vi "LS Durability Main ALTERNATE (FPGA).vi"() -> ()   [LabVIEW 2019]
uses:
  <vilib>/eio/EIONode/EIONode.xnode
  <vilib>/rvi/eio/common/nirviEmuTemplateMethod_errors.vi
  <vilib>/rvi/DataTransferAndStorage/Container/XNode/niFpgaContainer.xnode
  <vilib>/rvi/FIFO/Fifo_Resource/niFpgaFifoEmulationRefIn.vi
panel:
  out "FIFO microseconds":u32
  in  "Subtract Noise":bool
  out "Anomaly Array":fxp<+/-,29,18>[](array[numeric])
  in  "Enable2ndStepCheck":bool
  out "Anomaly Resamples":fxp<+/-,28,17>[](array[numeric])
  in  "Anomaly Threshold":fxp<+/-,28,17>=0.02978515625
  out "Bank2Active":bool
  out "Bank1Active":bool
  out "Bank2On":bool
  out "Bank1On":bool
  in  "Enable Readings":bool[](array[boolean])=[FALSE, FALSE, FALSE, FALSE, FALSE, FALSE, FALSE, FALSE, FALSE, FALSE, FALSE, FALSE]
  in  "Opens Resets":bool[](array[boolean])=[FALSE, FALSE, FALSE, FALSE, FALSE, FALSE, FALSE, FALSE, FALSE, FALSE, FALSE, FALSE]
  in  "Enable Opens":bool[](array[boolean])=[FALSE, FALSE, FALSE, FALSE, FALSE, FALSE, FALSE, FALSE, FALSE, FALSE, FALSE, FALSE]
  out "Opens Detected":u16[](array[numeric])
  out "Opens Loop Time (usec)":u32=1000
  in  "Bank2(Pulse/Const)":bool
  in  "Bank2Const(On/Off)":bool
  out "Anomalies (Last Cycle)":i32[](array[numeric])
  out "Cycle Starts":bool[](array[boolean])
  out "Anomalies (Total)":i32[](array[numeric])
  out "Anomalies/Cycle":i32[](array[numeric])
  in  "Normal Steps":u32=98
  out "Cycles":u32[](array[numeric])
  out "Anomaly Loop Time (usec)":u32=1000
  out "Steps":u32[](array[numeric])
  in  "Step Threshold":fxp<+/-,28,17>=0.02978515625
  in  "Enable Anomalies":bool[](array[boolean])=[FALSE, FALSE, FALSE, FALSE, FALSE, FALSE, FALSE, FALSE, FALSE, FALSE, FALSE, FALSE]
  in  "Anomaly Resets":bool[](array[boolean])=[FALSE, FALSE, FALSE, FALSE, FALSE, FALSE, FALSE, FALSE, FALSE, FALSE, FALSE, FALSE]
  in  "Bank1Const(On/Off)":bool
  in  "Bank1(Pulse/Const)":bool
  in  "PWM Period (Ticks)":u32=4000000
  in  "Duty (Ticks)":i32=2000000
  in  "Invert PWM?":bool=TRUE
  in  "Cycle Resets":bool[](array[boolean])=[FALSE, FALSE, FALSE, FALSE, FALSE, FALSE, FALSE, FALSE, FALSE, FALSE, FALSE, FALSE]
  in  "Points to Avg":i32=20
  in  "Enable Cycles":bool[](array[boolean])=[FALSE, FALSE, FALSE, FALSE, FALSE, FALSE, FALSE, FALSE, FALSE, FALSE, FALSE, FALSE]
  out "Total Cycles":u32[](array[numeric])
  in  "Cycle Threshold":fxp<+/-,28,17>=1.2001953125
  out "AI Avg Loop Time (usec)":u32=1000
  out "Analog Inputs":fxp<+/-,28,17>[](array[numeric])
  out "AI Loop Time (usec)":u32=70
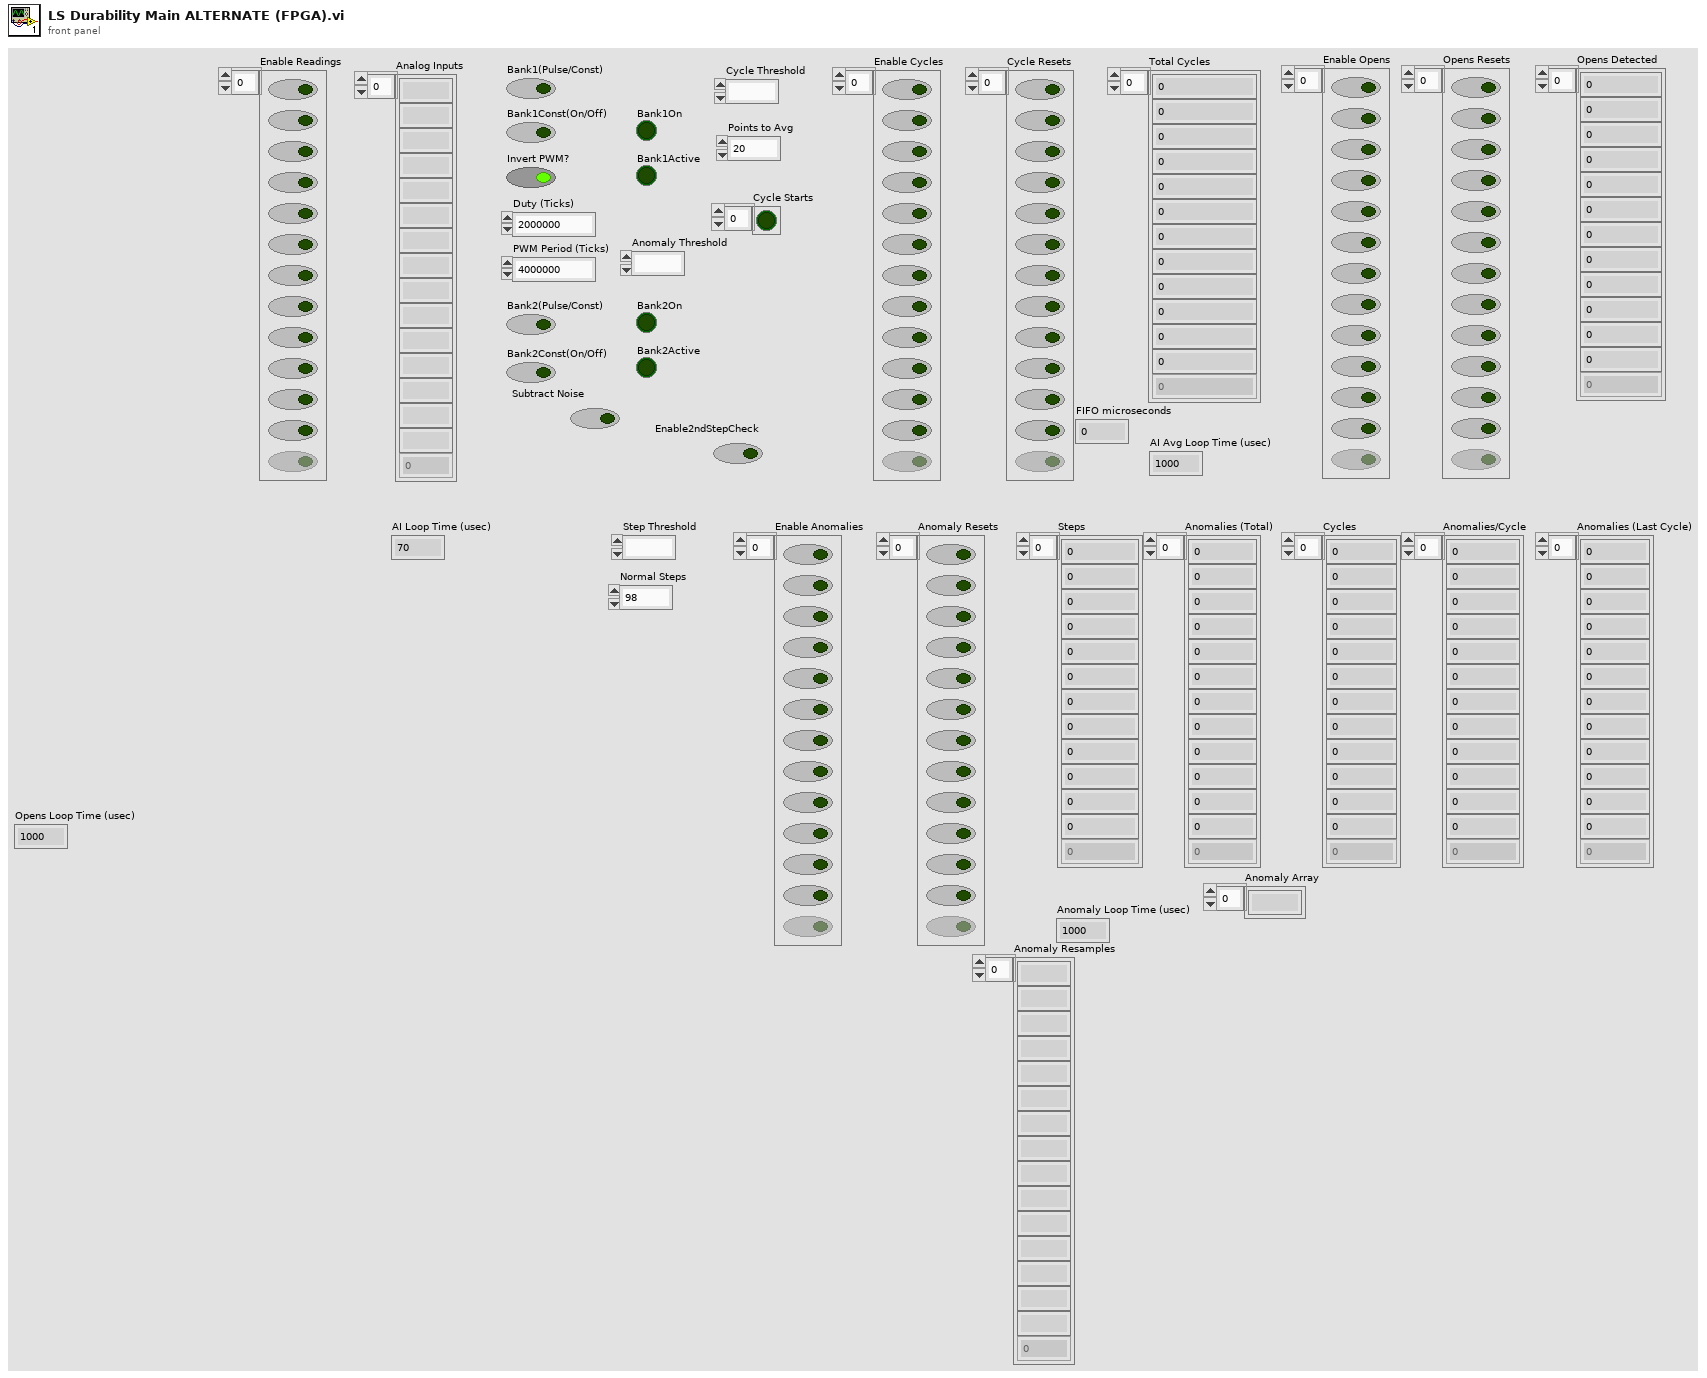
[diagram p1: front panel]
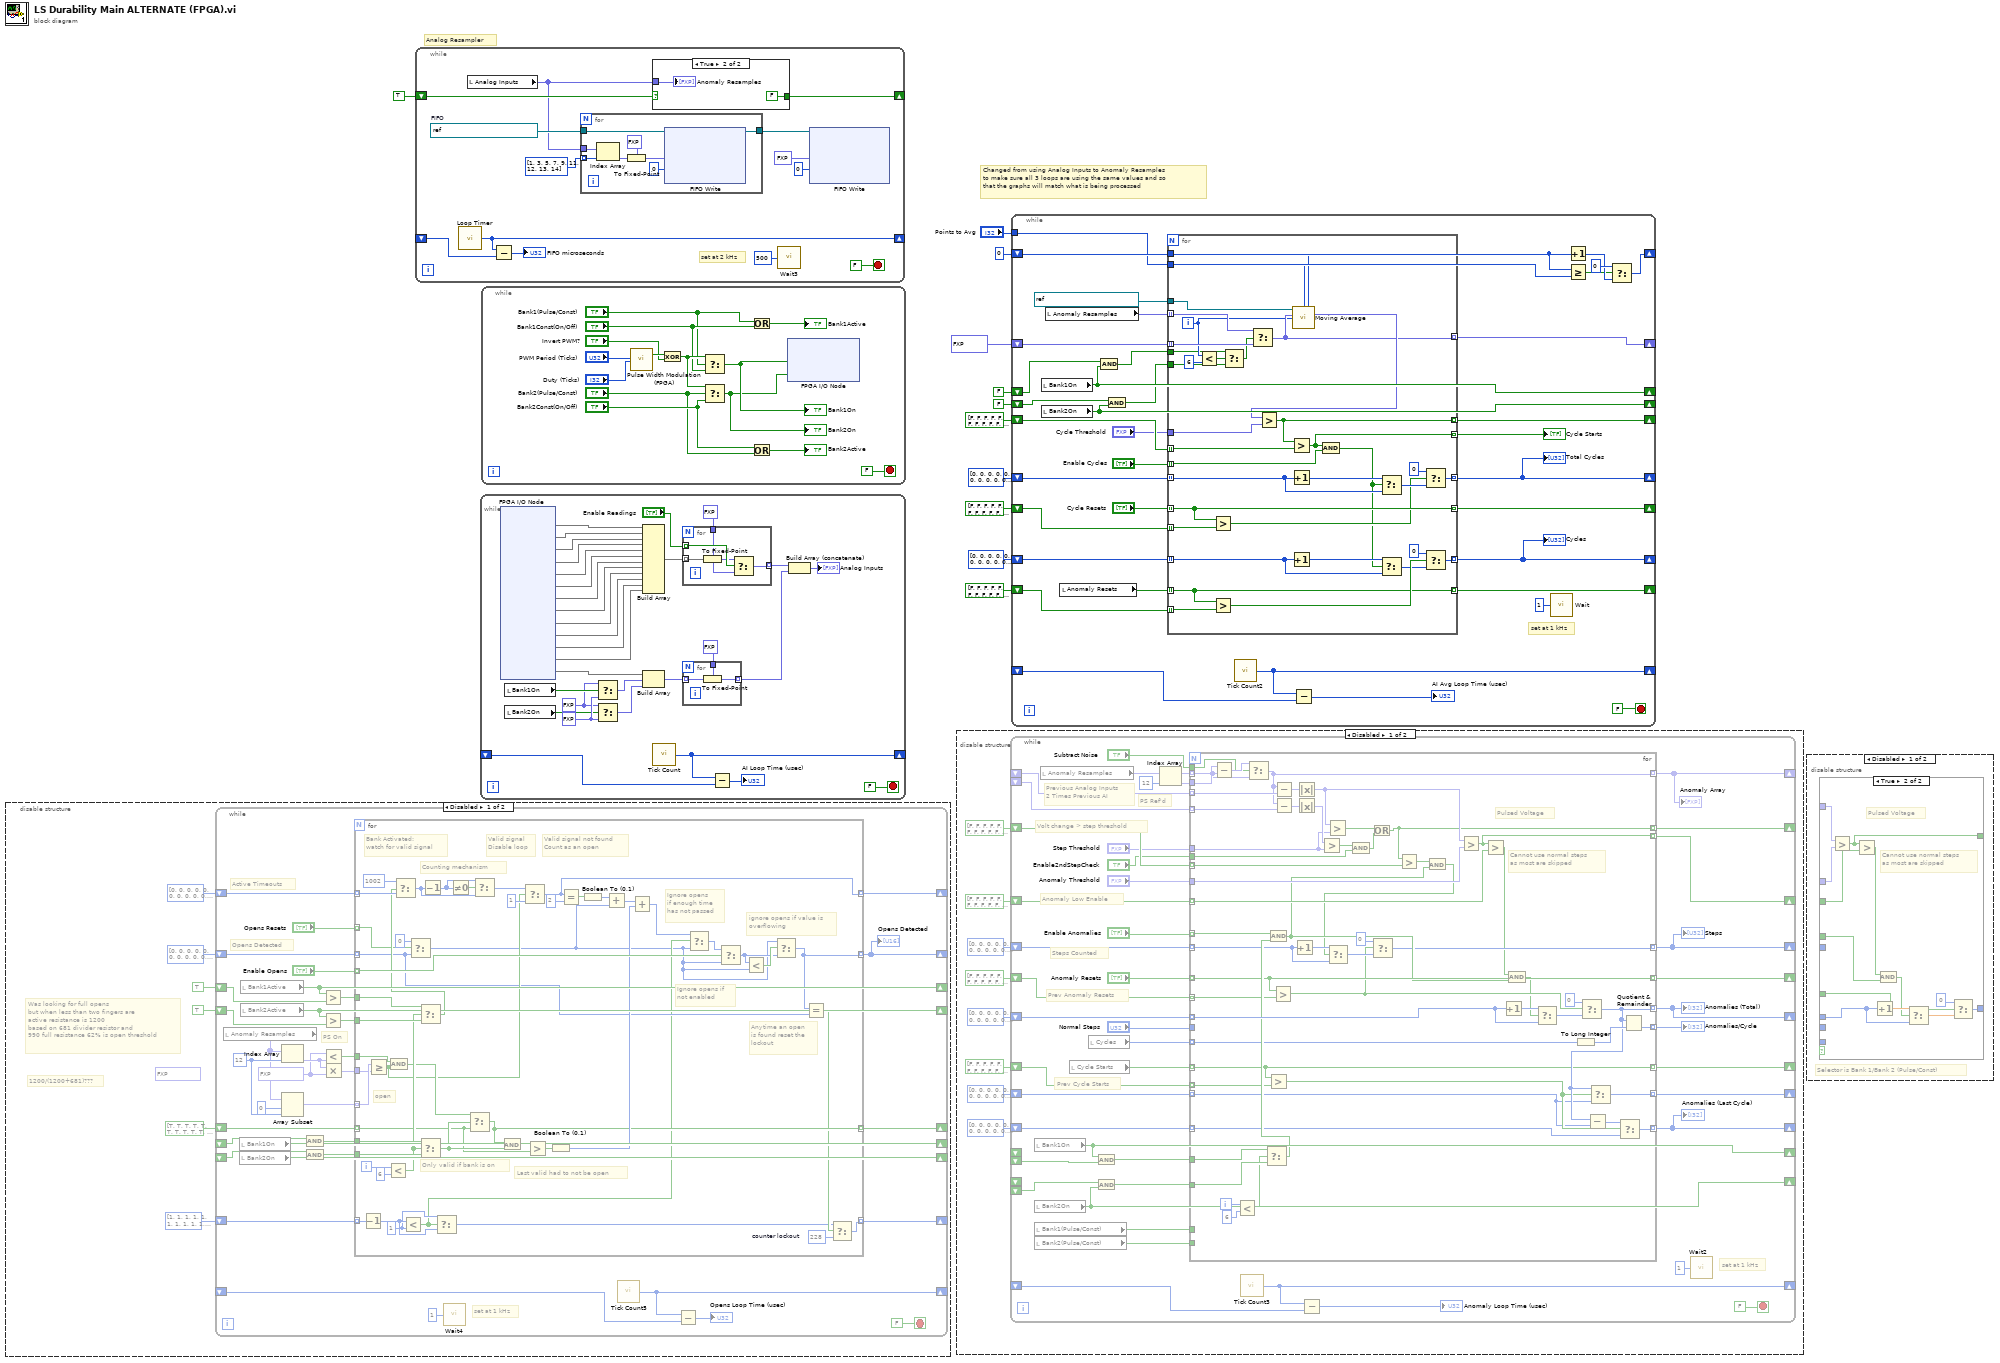
[diagram p0: block diagram]
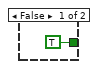
[diagram p4: hidden frame]
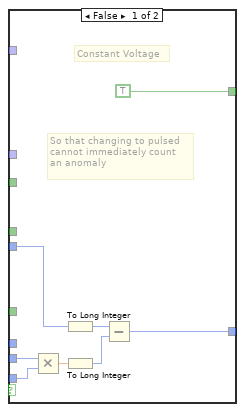
[diagram p5: hidden frame]
diagram:
  # "Changed from using Analog Inputs to Anomaly Resamples\nto make sure all 3 loops are using the same values and so\nthat the graphs will match what is being processed"
  # "Analog Resampler"
  n1 = disable-structure shown="Disabled" {
    frame Disabled {
      (unwired) fxp<+,8,0> 0.94921875
      # "1200/(1200+681)???"
      # "Was looking for full opens\nbut when less than two fingers are\nactive resistance is 1200\nbased on 681 divider resistor and\n990 full resistance 62% is open threshold"
      n2 = while {
        shift-right: [w50] -> _
        shift-left: _ -> [w49]
        shift-right: [w21] -> _
        shift-left: u8[] [0, 0, 0, 0, 0, 0, 0, 0, 0, 0, 0, 0] -> [w45]
        shift-right: [w30] -> _
        shift-left: u16[] [0, 0, 0, 0, 0, 0, 0, 0, 0, 0, 0, 0] -> [w31]
        shift-right: [w37] -> _
        shift-left: bool[] [TRUE, TRUE, TRUE, TRUE, TRUE, TRUE, TRUE, TRUE, TRUE, TRUE, TRUE, TRUE] -> [w36]
        shift-right: [w35] -> _
        shift-left: TRUE ("Bank2Active") -> [w33]
        shift-right: [w34] -> _
        shift-left: TRUE ("Bank1Active") -> [w32]
        shift-right: [w24] -> _
        shift-left: _ -> [w22]
        shift-right: [w25] -> _
        shift-left: _ -> [w23]
        shift-right: [w19] -> _
        shift-left: u16[] [1, 1, 1, 1, 1, 1, 1, 1, 1, 1, 1, 1] -> [w20]
        stop <- FALSE stop-if-true
        w38 = fxp<+,8,0> 0.62109375
        w47 = 12 ("length")
        # "Opens Detected"
        # "Active Timeouts"
        # "PS On"
        # "set at 1 kHz"
        n3 = local read "Anomaly Resamples"() -> (w18:fxp<+/-,28,17>[])
        n4 = local read "Bank1On"() -> (w25:bool)
        n5 = local read "Bank2On"() -> (w24:bool)
        n6 = local read "Bank1Active"() -> (w34:bool)
        n7 = local read "Bank2Active"() -> (w35:bool)
        n8 = Index Array(array=w18, index=w47) -> (element=w39:fxp<+/-,28,17>)
        n9 = Array Subset(array=w18, index=0, length=w47) -> (w40:fxp<+/-,28,17>[])
        n10 = And(x=w23, y=w25) -> (x .and. y?=w27:bool)
        n11 = And(x=w22, y=w24) -> (x .and. y?=w26:bool)
        n12 = Greater?(x=w34, y=w32) -> (0:w44:bool)
        n13 = Greater?(x=w35, y=w33) -> (0:w43:bool)
        n14 = Less?(x=w38, y=w39) -> (x < y?=w42:bool)
        n15 = Multiply(x=w39, y=w38) -> (x*y=w41:fxp<+/-,36,17>)
        n16 = for {
          tunnel: w27 -> [w99]
          tunnel: w26 -> [w98]
          tunnel: w44 -> [w96]
          tunnel: w43 -> [w97]
          tunnel: w45 -> [w57] mode=indexing
          tunnel: w31 -> [w84] mode=indexing
          tunnel: "Opens Resets" -> [w68] mode=indexing
          tunnel: "Enable Opens" -> [w82] mode=indexing
          tunnel: [w58] -> w21 mode=indexing
          tunnel: w41 -> [w79]
          tunnel: w40 -> [w80] mode=indexing
          tunnel: w42 -> [w78]
          tunnel: [w69] -> w37 mode=indexing
          tunnel: w36 -> [w74] mode=indexing
          tunnel: [w72] -> w30 mode=indexing
          tunnel: w20 -> [w63] mode=indexing
          tunnel: [w59] -> w19 mode=indexing
          i -> [w101]
          w60 = u16 228  # counter lockout
          w64 = u16 1 ("y")
          # "Ignore opens if\nnot enabled"
          # "Ignore opens\nif enough time\nhas not passed"
          # "Anytime an open\nis found reset the\nlockout"
          # "ignore opens if value is\noverflowing"
          # "Last valid had to not be open"
          # "Only valid if bank is on"
          # "open"
          # "Valid signal not found\nCount as an open"
          # "Valid signal\nDisable loop"
          # "Counting mechanism"
          # "Bank Activated:\nwatch for valid signal"
          n17 = Decrement(x=w63) -> (x-1=w65:u16)
          n18 = Greater Or Equal?(x=w80, y=w79) -> (x >= y?=w71:bool)
          n19 = Less?(x=w101, y=6) -> (x < y?=w95:bool)
          n20 = And(x=w78, y=w71) -> (x .and. y?=w77:bool)
          n21 = Less?(x=w65, y=w64) -> (x < y?=w54:bool)
          n22 = Select(t=u16 0, s=w68, f=w57) -> (s? t:f=w53:u16)
          n23 = Select(t=w96, s=w95, f=w97) -> (s? t:f=w81:bool)
          n24 = Select(t=u16 1002, s=w81, f=w84) -> (s? t:f=w83:u16)
          n25 = Select(t=w99, s=w95, f=w98) -> (s? t:f=w76:bool)
          n26 = Decrement(x=w83) -> (x-1=w88:u16)
          n27 = Select(t=w64, s=w54, f=w65) -> (s? t:f=w61:u16)
          n28 = Not Equal To 0?(x=w88) -> (x != 0?=w87:bool)
          n29 = Select(t=w77, s=w76, f=w74) -> (s? t:f=w69:bool)
          n30 = Select(t=w88, s=w87, f=w83) -> (s? t:f=w89:u16)
          n31 = And(x=w69, y=w76) -> (x .and. y?=w70:bool)
          n32 = Select(t=w89, s=w71, f=u16 1) -> (s? t:f=w72:u16)
          n33 = Greater?(x=w70, y=w74) -> (0:w75:bool)
          n34 = Boolean To (0,1)(Boolean=w75) -> (0, 1=w73:i16)
          n35 = Equal?(x=w72, y=u16 2) -> (x = y?=w91:bool)
          n36 = Boolean To (0,1)(Boolean=w91) -> (0, 1=w92:i16)
          n37 = Add(x=w92, y=w53) -> (x+y=w93:u16)
          n38 = Add(x=w93, y=w73) -> (x+y=w55:u16)
          n39 = Select(t=w55, s=w54, f=w53) -> (s? t:f=w56:u16)
          n40 = Select(t=w56, s=w82, f=w53) -> (s? t:f=w66:u16)
          n41 = Less?(x=w66, y=w53) -> (x < y?=w67:bool)
          n42 = Select(t=w53, s=w67, f=w66) -> (s? t:f=w58:u16)
          n43 = Equal?(x=w58, y=w57) -> (x = y?=w62:bool)
          n44 = Select(t=w61, s=w62, f=w60) -> (s? t:f=w59:u16)
        }
        "Opens Detected" <- w21
        n45 = call "Wait4"("Count(mSec)"=u32 1) -> ()  [unwired: 1 out]
        n46 = call "Tick Count5"() -> ("Tick Count(uSec)"=w50:u32)
        n47 = Subtract(x=w50, y=w49) -> (x-y=→"Opens Loop Time (usec)":u32)
      }
    }
    frame Enabled {
    }
  }
  n48 = while {
    shift-right: [w113] -> _
    shift-left: TRUE -> [w111]
    shift-right: [w105] -> _
    shift-left: _ -> [w104]
    stop <- FALSE stop-if-true
    w110 = refnum<k21> "One Hour Analog Data"  # FIFO
    # "set at 2 kHz"
    n49 = call "Loop Timer"() -> ("Tick Count(uSec)"=w105:u32)  [unwired: 1 in]
    n50 = local read "Analog Inputs"() -> (w109:fxp<+/-,28,17>[])
    n51 = Subtract(x=w105, y=w104) -> (x-y=→"FIFO microseconds":u32)
    n52 = for {
      tunnel: w110 -> [w122]
      tunnel: w109 -> [w117]
      tunnel: [w118] -> w108
      tunnel: i32[] [1, 3, 5, 7, 9, 11, 12, 13, 14] -> [w115] mode=indexing
      n53 = Index Array(array=w117, index=w115) -> (element=w116:fxp<+/-,28,17>)
      n54 = To Fixed-Point(fixed-point type=fxp<+/-,18,5> 0.0 ("AI0"), number=w116) -> (fixed-point=w121:fxp<+/-,18,5>)
      n55 = xnode ("FIFO Write")("Element"=w121, "Timeout"=0, "FIFO In"=w122) -> ("FIFO Out"=w118:refnum<k21>)  [unwired: 1 out]
    }
    n56 = case shown="True" w111 {
      tunnel: w109 -> [_ w125]
      tunnel: [TRUE FALSE] -> w113
      frame False {
      }
      frame True {
        "Anomaly Resamples" <- w125
      }
    }
    n57 = call "Wait3"("Count(uSec)"=u32 500 ("Count(mSec)")) -> ()  [unwired: 1 out]
    n58 = xnode ("FIFO Write")("Element"=fxp<+/-,18,5> -15.0 ("AI0"), "Timeout"=0, "FIFO In"=w108) -> ()  [unwired: 2 out]
  }
  n59 = while {
    shift-right: [w155] -> _
    shift-left: _ -> [w154]
    stop <- FALSE stop-if-true
    w128 = fxp<+/-,24,5> 1.0 ("AI13")
    w131 = fxp<+/-,24,5> 0.0 ("AI13")
    n60 = xnode "FPGA I/O Node"() -> ("AI0"=w152, "AI1"=w151, "AI2"=w150, "AI3"=w149, "AI4"=w148, "AI5"=w147, "AI6"=w146, "AI7"=w145, "AI8"=w144, "AI9"=w143, "AI10"=w142, "AI11"=w141, "AI12"=w138)  [unwired: 13 in, 13 out]
    n61 = local read "Bank1On"() -> (w130:bool)
    n62 = local read "Bank2On"() -> (w129:bool)
    n63 = Select(t=w128, s=w130, f=w131) -> (s? t:f=w127:fxp<+/-,24,5>)
    n64 = Select(t=w128, s=w129, f=w131) -> (s? t:f=w126:fxp<+/-,24,5>)
    n65 = Build Array(w152, w151, w150, w149, w148, w147, w146, w145, w144, w143, w142, w141) -> (w140:void[])
    n66 = Build Array(w138, w127, w126) -> (w136:fxp<+/-,24,5>[])
    n67 = call "Tick Count"() -> ("Tick Count(uSec)"=w155:u32)
    n68 = for {
      tunnel: w140 -> [w164] mode=indexing
      tunnel: fxp<+/-,28,17> 0.0 ("AI0") -> [w161]
      tunnel: [w160] -> w134 mode=indexing
      tunnel: "Enable Readings" -> [w163] mode=indexing
      n69 = To Fixed-Point(fixed-point type=w161, number=w164) -> (fixed-point=w162:fxp<+/-,28,17>)
      n70 = Select(t=w162, s=w163, f=w161) -> (s? t:f=w160:fxp<+/-,28,17>)
    }
    n71 = for {
      tunnel: w136 -> [w159] mode=indexing
      tunnel: fxp<+/-,28,17> 0.0 ("AI0") -> [w158]
      tunnel: [w157] -> w135 mode=indexing
      n72 = To Fixed-Point(fixed-point type=w158, number=w159) -> (fixed-point=w157:fxp<+/-,28,17>)
    }
    n73 = Subtract(x=w155, y=w154) -> (x-y=→"AI Loop Time (usec)":u32)
    n74 = Build Array (concatenate)(w134, w135) -> (→"Analog Inputs":fxp<+/-,28,17>[])
  }
  n75 = while {
    stop <- FALSE stop-if-true
    n76 = call "Pulse Width Modulation (FPGA).vi"("PWM Period (Ticks)"="PWM Period (Ticks)", "PWM Duty Cycle (Ticks)"="Duty (Ticks)") -> ("PWM DO"=w175:bool)  [unwired: 14 in, 3 out]
    n77 = Exclusive Or(1:"Invert PWM?", 2:w175) -> (0:w173:bool)
    n78 = Select(t=w173, s="Bank1(Pulse/Const)", f="Bank1Const(On/Off)") -> (s? t:f=w172:bool)
    "Bank1On" <- w172
    n79 = Select(t=w173, s="Bank2(Pulse/Const)", f="Bank2Const(On/Off)") -> (s? t:f=w171:bool)
    "Bank2On" <- w171
    n80 = Or(x="Bank1(Pulse/Const)", y="Bank1Const(On/Off)") -> (x .or. y?=→"Bank1Active":bool)
    n81 = Or(x="Bank2Const(On/Off)", y="Bank2(Pulse/Const)") -> (x .or. y?=→"Bank2Active":bool)
    n82 = xnode "FPGA I/O Node"("RMC/DIO0"=w172, "RMC/DIO1"=w171) -> ()  [unwired: 3 in, 3 out]
  }
  n83 = disable-structure shown="Disabled" {
    frame Disabled {
      n84 = while {
        shift-right: [w228] -> _
        shift-left: _ -> [w227]
        shift-right: [w220] -> _
        shift-left: bool[] [FALSE, FALSE, FALSE, FALSE, FALSE, FALSE, FALSE, FALSE, FALSE, FALSE, FALSE, FALSE] -> [w219]
        shift-right: [w217] -> _
        shift-left: u32[] [0, 0, 0, 0, 0, 0, 0, 0, 0, 0, 0, 0] -> [w216]
        shift-right: [w215] -> _
        shift-left: bool[] [FALSE, FALSE, FALSE, FALSE, FALSE, FALSE, FALSE, FALSE, FALSE, FALSE, FALSE, FALSE] -> [w212]
        shift-right: [w222] -> _
        shift-left: _ -> [w221]
        shift-right: [w209] -> _
        shift-left: bool[] [FALSE, FALSE, FALSE, FALSE, FALSE, FALSE, FALSE, FALSE, FALSE, FALSE, FALSE, FALSE] -> [w208]
        shift-right: [w207] -> _
        shift-left: i32[] [0, 0, 0, 0, 0, 0, 0, 0, 0, 0, 0, 0] -> [w205]
        shift-right: [w206] -> _
        shift-left: i32[] [0, 0, 0, 0, 0, 0, 0, 0, 0, 0, 0, 0] -> [w204]
        shift-right: [w196] -> _
        shift-left: _ -> [_]
        shift-right: [w223] -> _
        shift-left: _ -> [_]
        shift-right: [w201] -> _
        shift-left: i32[] [0, 0, 0, 0, 0, 0, 0, 0, 0, 0, 0, 0] -> [w200]
        shift-right: [w197] -> _
        shift-left: bool[] [FALSE, FALSE, FALSE, FALSE, FALSE, FALSE, FALSE, FALSE, FALSE, FALSE, FALSE, FALSE] -> [w198]
        shift-left: _ -> [w194]
        shift-left: _ -> [w195]
        shift-left: _ -> [w192]
        stop <- FALSE stop-if-true
        # "PS Ref'd"
        # "Anomaly Low Enable"
        # "Prev Cycle Starts"
        # "Prev Anomaly Resets"
        # "Steps Counted"
        # "Volt change > step threshold"
        # "Previous Analog Inputs\n2 Times Previous AI"
        # "set at 1 kHz"
        n85 = local read "Bank1On"() -> (w196:bool)
        n86 = local read "Bank2On"() -> (w223:bool)
        n87 = local read "Bank1(Pulse/Const)"() -> (w203:bool)
        n88 = local read "Bank2(Pulse/Const)"() -> (w202:bool)
        n89 = local read "Anomaly Resamples"() -> (w190:fxp<+/-,28,17>[])
        n90 = local read "Cycle Starts"() -> (w210:bool[])
        n91 = local read "Cycles"() -> (w211:u32[])
        n92 = And(x=w196, y=w195) -> (x .and. y?=w225:bool)
        n93 = And(x=w194, y=w223) -> (x .and. y?=w224:bool)
        n94 = Index Array(array=w190, index=12) -> (element=w189:fxp<+/-,28,17>)
        n95 = for {
          tunnel: w190 -> [w233] mode=indexing
          tunnel: [w240] -> w220 mode=indexing
          tunnel: w219 -> [w261] mode=indexing
          tunnel: w216 -> [w254] mode=indexing
          tunnel: [w253] -> w217 mode=indexing
          tunnel: "Step Threshold" -> [w242]
          tunnel: "Enable Anomalies" -> [w280] mode=indexing
          tunnel: "Anomaly Resets" -> [w263] mode=indexing
          tunnel: [w263] -> w215 mode=indexing
          tunnel: w212 -> [w264] mode=indexing
          tunnel: [w234] -> w222 mode=indexing
          tunnel: w221 -> [w281] mode=indexing
          tunnel: "Normal Steps" -> [_]
          tunnel: w211 -> [w271] mode=indexing
          tunnel: [w270] -> w213 mode=indexing
          tunnel: [w272] -> w201 mode=indexing
          tunnel: w210 -> [w266] mode=indexing
          tunnel: [w266] -> w209 mode=indexing
          tunnel: w208 -> [w267] mode=indexing
          tunnel: [w269] -> w207 mode=indexing
          tunnel: w205 -> [w252] mode=indexing
          tunnel: [w268] -> w206 mode=indexing
          tunnel: w204 -> [w251] mode=indexing
          tunnel: w225 -> [w288]
          tunnel: w224 -> [w287]
          tunnel: w203 -> [_]
          tunnel: w202 -> [_]
          tunnel: w200 -> [w283] mode=indexing
          tunnel: "Anomaly Threshold" -> [w277]
          tunnel: w198 -> [w276] mode=indexing
          tunnel: [w275] -> w197 mode=indexing
          tunnel: w192 -> [w244] mode=indexing
          tunnel: "Enable2ndStepCheck" -> [w237]
          tunnel: w189 -> [w236]
          tunnel: "Subtract Noise" -> [w232]
          i -> [w286]
          # "Cannot use normal steps\nas most are skipped"
          # "Pulsed Voltage"
          n96 = Subtract(x=w236, y=w233) -> (x-y=w235:fxp<+/-,29,18>)
          n97 = Less?(x=w286, y=6) -> (x < y?=w284:bool)
          n98 = Select(t=w235, s=w232, f=w233) -> (s? t:f=w234:fxp<+/-,29,18>)
          n99 = Select(t=w288, s=w284, f=w287) -> (s? t:f=w279:bool)
          n100 = And(x=w280, y=w279) -> (x .and. y?=w260:bool)
          n101 = Greater?(x=w266, y=w267) -> (0:w265:bool)
          n102 = Greater?(x=w263, y=w264) -> (0:w256:bool)
          n103 = Subtract(x=w234, y=w281) -> (x-y=w282:fxp<+/-,30,19>)
          n104 = Subtract(x=w234, y=w244) -> (x-y=w245:fxp<+/-,30,19>)
          n105 = Increment(x=w254) -> (x+1=w257:u32)
          n106 = Absolute Value(x=w282) -> (abs(x)=w278:fxp<+,29,18>)
          n107 = Absolute Value(x=w245) -> (abs(x)=w243:fxp<+,29,18>)
          n108 = Greater?(x=w243, y=w242) -> (0:w239:bool)
          n109 = Greater?(x=w278, y=w242) -> (0:w241:bool)
          n110 = And(x=w239, y=w237) -> (x .and. y?=w238:bool)
          n111 = Or(x=w241, y=w238) -> (x .or. y?=w240:bool)
          n112 = Greater?(x=w240, y=w261) -> (0:w262:bool)
          n113 = And(x=w262, y=w260) -> (x .and. y?=w255:bool)
          n114 = Select(t=w257, s=w255, f=w254) -> (s? t:f=w258:u32)
          n115 = Select(t=u32 0, s=w256, f=w258) -> (s? t:f=w253:u32)
          n116 = Greater?(x=w278, y=w277) -> (0:w275:bool)
          n117 = Greater?(x=w275, y=w276) -> (0:w246:bool)
          n118 = Increment(x=w283) -> (x+1=w248:i32)
          n119 = And(x=w246, y=w260) -> (x .and. y?=w247:bool)
          n120 = Select(t=w248, s=w247, f=w283) -> (s? t:f=w249:i32)
          n121 = To Long Integer(number=w271) -> (32bit integer=w273:i32)
          n122 = Select(t=0, s=w256, f=w249) -> (s? t:f=w272:i32)
          n123 = Subtract(x=w272, y=w252) -> (x-y=w274:i32)
          n124 = Select(t=w272, s=w265, f=w252) -> (s? t:f=w269:i32)
          n125 = Select(t=w274, s=w265, f=w251) -> (s? t:f=w268:i32)
          n126 = Quotient & Remainder(x=w272, y=w273) -> (floor(x/y)=w270:i32)  [unwired: 1 out]
        }
        "Steps" <- w217
        "Anomalies/Cycle" <- w213
        "Anomalies (Total)" <- w201
        "Anomalies (Last Cycle)" <- w206
        "Anomaly Array" <- w222
        n127 = call "Tick Count3"() -> ("Tick Count(uSec)"=w228:u32)
        n128 = Subtract(x=w228, y=w227) -> (x-y=→"Anomaly Loop Time (usec)":u32)
        n129 = call "Wait2"("Count(mSec)"=u32 1) -> ()  [unwired: 1 out]
      }
    }
    frame Enabled {
    }
  }
  n130 = while {
    shift-right: [w318] -> _
    shift-left: 0 ("Moving Point Index") -> [w319]
    shift-right: [w315] -> _
    shift-left: _ -> [w314]
    shift-right: [w313] -> _
    shift-left: bool[] [FALSE, FALSE, FALSE, FALSE, FALSE, FALSE, FALSE, FALSE, FALSE, FALSE, FALSE, FALSE] -> [w312]
    shift-right: [w310] -> _
    shift-left: u32[] [0, 0, 0, 0, 0, 0, 0, 0, 0, 0, 0, 0] -> [w311]
    tunnel: "Points to Avg" -> [w307]
    shift-right: [w305] -> _
    shift-left: bool[] [FALSE, FALSE, FALSE, FALSE, FALSE, FALSE, FALSE, FALSE, FALSE, FALSE, FALSE, FALSE] -> [w304]
    shift-right: [w299] -> _
    shift-left: u32[] [0, 0, 0, 0, 0, 0, 0, 0, 0, 0, 0, 0] -> [w301]
    shift-right: [w302] -> _
    shift-left: bool[] [FALSE, FALSE, FALSE, FALSE, FALSE, FALSE, FALSE, FALSE, FALSE, FALSE, FALSE, FALSE] -> [w303]
    shift-right: [w295] -> _
    shift-left: FALSE -> [w293]
    shift-right: [w291] -> _
    shift-left: FALSE -> [w292]
    shift-right: [w296] -> _
    shift-left: fxp<+/-,28,17>[] [0.0, 0.0, 0.0, 0.0, 0.0, 0.0, 0.0, 0.0, 0.0, 0.0, 0.0, 0.0] ("Analog Inputs") -> [w297]
    stop <- FALSE stop-if-true
    # "set at 1 kHz"
    n131 = local read "Bank1On"() -> (w295:bool)
    n132 = local read "Bank2On"() -> (w291:bool)
    n133 = local read "Anomaly Resamples"() -> (w289:fxp<+/-,28,17>[])
    n134 = local read "Anomaly Resets"() -> (w300:bool[])
    n135 = And(x=w293, y=w295) -> (x .and. y?=w294:bool)
    n136 = And(x=w292, y=w291) -> (x .and. y?=w290:bool)
    n137 = for {
      tunnel: w319 -> [w357]
      tunnel: w307 -> [w358]
      tunnel: w289 -> [w333] mode=indexing
      tunnel: refnum<k21> "Running Avg Memory" ("Memory") -> [w359]
      tunnel: [w356] -> w313 mode=indexing
      tunnel: w312 -> [w355] mode=indexing
      tunnel: w311 -> [w353] mode=indexing
      tunnel: [w345] -> w310 mode=indexing
      tunnel: "Cycle Threshold" -> [w352]
      tunnel: "Enable Cycles" -> [w351] mode=indexing
      tunnel: "Cycle Resets" -> [w350] mode=indexing
      tunnel: [w350] -> w305 mode=indexing
      tunnel: w304 -> [w349] mode=indexing
      tunnel: w301 -> [w338] mode=indexing
      tunnel: [w344] -> w299 mode=indexing
      tunnel: w300 -> [w339] mode=indexing
      tunnel: [w339] -> w302 mode=indexing
      tunnel: w303 -> [w340] mode=indexing
      tunnel: [w336] -> w298 mode=indexing
      tunnel: w297 -> [w334] mode=indexing
      tunnel: [w332] -> w296 mode=indexing
      tunnel: w294 -> [w327]
      tunnel: w290 -> [w326]
      i -> [w329]
      n138 = Less?(x=w329, y=6) -> (x < y?=w330:bool)
      n139 = Greater?(x=w350, y=w349) -> (0:w347:bool)
      n140 = Greater?(x=w339, y=w340) -> (0:w342:bool)
      n141 = Select(t=w327, s=w330, f=w326) -> (s? t:f=w328:bool)
      n142 = Select(t=w333, s=w328, f=w334) -> (s? t:f=w332:fxp<+/-,28,17>)
      n143 = Increment(x=w353) -> (x+1=w354:u32)
      n144 = Increment(x=w338) -> (x+1=w337:u32)
      n145 = call "Moving Average.vi"("Memory In"=w359, "N (# of Ave Pts 127 max)"=w358, "Moving Point Index"=w357, "Data IN"=w332, "Channel#"=w329) -> ("Averaged Data"=w335:fxp<+/-,28,17>)  [unwired: 10 in]
      n146 = Greater?(x=w335, y=w352) -> (0:w356:bool)
      n147 = Greater?(x=w356, y=w355) -> (0:w336:bool)
      n148 = And(x=w336, y=w351) -> (x .and. y?=w325:bool)
      n149 = Select(t=w354, s=w325, f=w353) -> (s? t:f=w348:u32)
      n150 = Select(t=w337, s=w325, f=w338) -> (s? t:f=w341:u32)
      n151 = Select(t=u32 0, s=w347, f=w348) -> (s? t:f=w345:u32)
      n152 = Select(t=u32 0, s=w342, f=w341) -> (s? t:f=w344:u32)
    }
    "Total Cycles" <- w310
    "Cycles" <- w299
    "Cycle Starts" <- w298
    n153 = call "Tick Count2"() -> ("Tick Count(uSec)"=w315:u32)
    n154 = Subtract(x=w315, y=w314) -> (x-y=→"AI Avg Loop Time (usec)":u32)
    n155 = call "Wait"("Count(mSec)"=u32 1) -> ()  [unwired: 1 out]
    n156 = Increment(x=w319) -> (x+1=w321:i32)
    n157 = Greater Or Equal?(x=w319, y=w307) -> (x >= y?=w320:bool)
    n158 = Select(t=0, s=w320, f=w321) -> (s? t:f=w318:i32)
  }
  n159 = disable-structure shown="Disabled" {
    frame Disabled {
      # "Selector is Bank 1/Bank 2 (Pulse/Const)"
      n160 = case shown="True" {
        selector: _ -> [_ _]
        tunnel: _ -> [w367 _]
        tunnel: _ -> [w363 _]
        tunnel: [w362 w376] -> _
        tunnel: _ -> [w360 _]
        tunnel: _ -> [_ w377]
        tunnel: _ -> [_ w373]
        tunnel: _ -> [_ w374]
        tunnel: _ -> [_ w372]
        tunnel: _ -> [_ w371]
        tunnel: [TRUE w370] -> _
        tunnel: _ -> [_ w368]
        frame False {
          # "So that changing to pulsed\ncannot immediately count\nan anomaly"
          # "Constant Voltage"
          n161 = Multiply(x=w367, y=w363) -> (x*y=w366:dbl)
          n162 = To Long Integer(number=w360) -> (32bit integer=w365:i32)
          n163 = To Long Integer(number=w366) -> (32bit integer=w364:i32)
          n164 = Subtract(x=w365, y=w364) -> (x-y=w362:i32)
        }
        frame True {
          # "Cannot use normal steps\nas most are skipped"
          # "Pulsed Voltage"
          n165 = Greater?(x=w373, y=w372) -> (0:w370:bool)
          n166 = Greater?(x=w370, y=w371) -> (0:w369:bool)
          n167 = Increment(x=w377) -> (x+1=w378:dbl)
          n168 = And(x=w369, y=w374) -> (x .and. y?=w375:bool)
          n169 = Select(t=w378, s=w375, f=w377) -> (s? t:f=w379:dbl)
          n170 = Select(t=0, s=w368, f=w379) -> (s? t:f=w376:i32)
        }
      }
    }
    frame Enabled {
    }
  }
